vi "Write Input Registers1.vi"(8 "error in (no error)":errorcluster, 9 "register values":u16[](array[numeric]), 10 "starting address":u16, 11 "standard data model in":refnum<class "Standard Data Model1.lvclass">) -> (0 "error out":errorcluster, 3 "standard data model out":refnum<class "Standard Data Model1.lvclass">)   [LabVIEW 2021, in "NI_modbus_upd.lvlib" / "Standard Data Model1.lvclass"]
doc: "Writes the values of multiple input register values in series, starting at address M."
uses:
  Standard Data Model1.lvclass
  Standard Data Model1.lvclass/Standard Data Model1.ctl
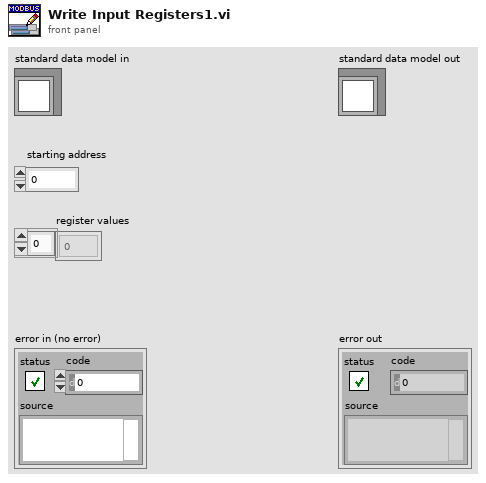
[diagram p1: front panel]
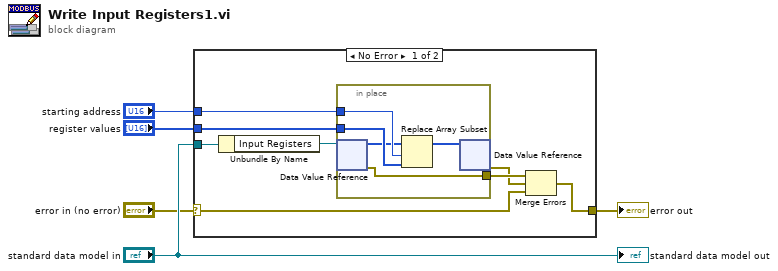
[diagram p0: block diagram]
diagram:
  n1 = case shown="No Error" "error in (no error)" {
    selector: "error in (no error)" -> [w6 w19]
    tunnel: "starting address" -> [w13 _]
    tunnel: "register values" -> [w12 _]
    tunnel: "standard data model in" -> [w11 _]
    tunnel: [w9 w19] -> w2
    frame No Error {
      n2 = Unbundle By Name(w11) -> ("Input Registers"=w10:refnum<data-value>)
      n3 = in-place {
        in-place-border: w13 -> [w18]
        in-place-border: w12 -> [w17]
        in-place-border: [w14] -> w8
        n4 = in-place-dvr #1(w10) -> (w16:u16[], w14:errorcluster)
        n5 = Replace Array Subset(array=w16, new element=w17, index=w18) -> (w15:u16[])
        n6 = in-place-dvr #1(w15) -> (w7:errorcluster)  [unwired: 1 out]
      }
      n7 = Merge Errors(w8, w7, w6) -> (w9:errorcluster)
    }
    frame Error {
    }
  }
  "error out" <- w2
  "standard data model out" <- "standard data model in"
